vi "Ball and Beam(No Low Pass Fifter)2.vi"() -> ()   [LabVIEW 2011]
uses:
  <vilib>/Utility/file.llb/Write To Spreadsheet File (DBL).vi
  Instance           1 41Saved   Ball and Beam(No Low Pass Fifter) .vi
  Instance           2 41Saved   Ball and Beam(No Low Pass Fifter) .vi
panel:
  in  "file path (dialog if empty)":path
  out "Theta Output":dbl
  out "X Error":dbl
  out "X Error":dbl(graph)=-0.6885397082002527
  in  "Theta Bound":dbl=3.0
  in  "Kp":dbl=0.5
  in  "Kd":dbl
  in  "X disire":dbl
  out "Vout":dbl
  in  "Vout Bound":dbl=4.5
  in  "Kp1":dbl=1.0
  in  "Sampling rate(Hz)":dbl=50.0
  out "Theta":dbl
  in  "t offset":dbl
  in  "t amp":dbl
  out "Position":dbl
  in  "x offset":dbl
  in  "x amp":dbl
  out "Theta voltage":dbl
  out "X voltage":dbl
  in  "stop":bool
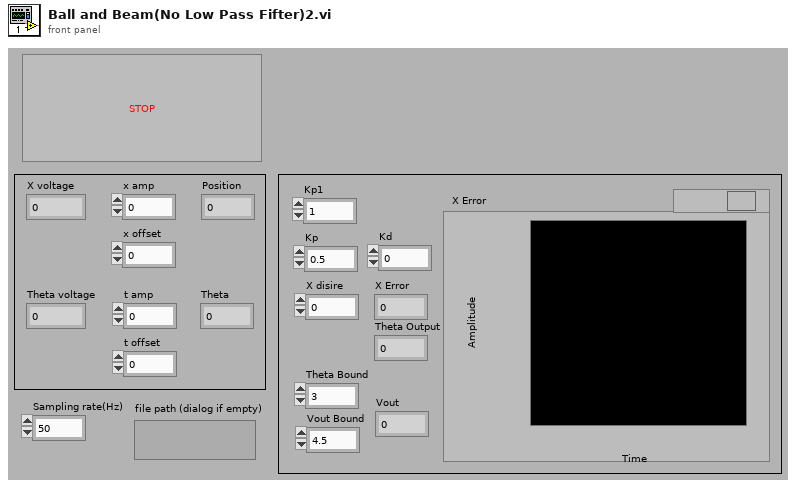
[diagram p1: front panel]
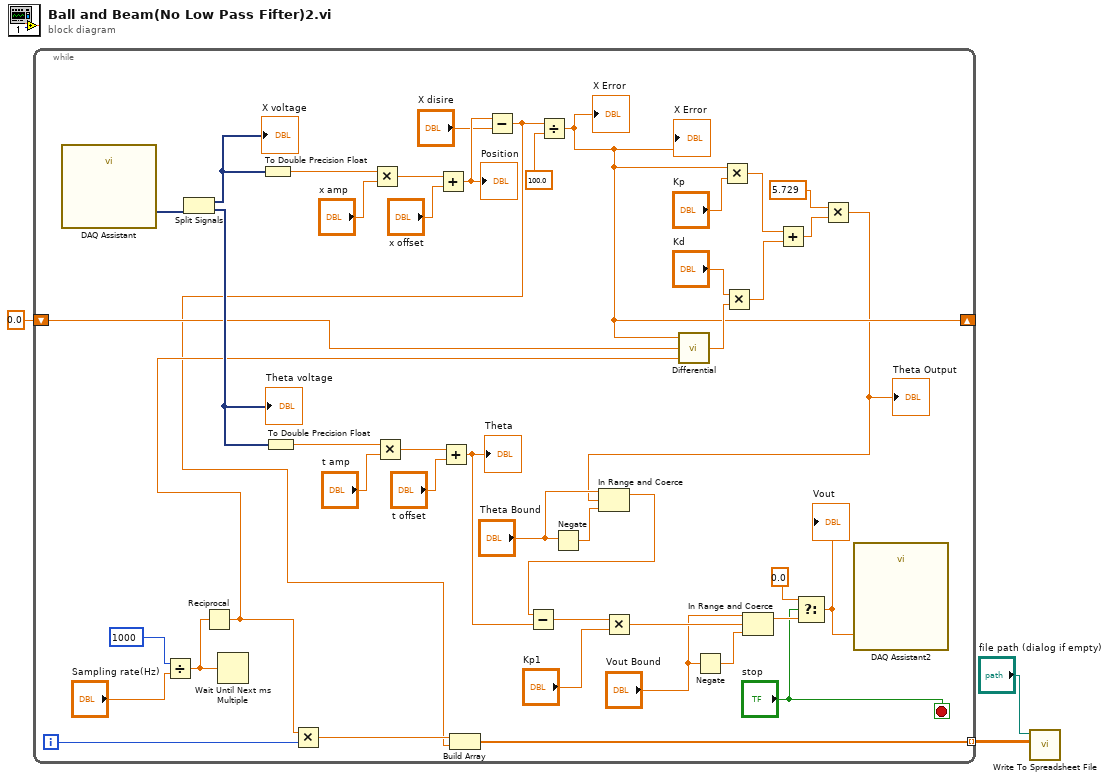
[diagram p0: block diagram]
diagram:
  n1 = while {
    shift-right: [w10] -> _
    shift-left: 0.0 -> [w19]
    tunnel: [w4] -> w2 mode=indexing
    i -> [w12]
    stop <- "stop" stop-if-true
    n2 = call "DAQ Assistant"() -> ("data"=w44:dynamicdata)  [unwired: 17 in, 2 out]
    n3 = Divide(x=1000, y="Sampling rate(Hz)") -> (x/y=w25:dbl)
    n4 = Split Signals(w44) -> (w43:dynamicdata, w38:dynamicdata)  [unwired: 2 in]
    "X voltage" <- w43
    "Theta voltage" <- w38
    n5 = Reciprocal(x=w25) -> (1/x=w11:dbl)
    n6 = Wait Until Next ms Multiple(millisecond multiple=w25) -> ()  [unwired: 1 out]
    n7 = To Double Precision Float(number=w43) -> (double precision float=w48:dbl)
    n8 = To Double Precision Float(number=w38) -> (double precision float=w42:dbl)
    n9 = Multiply(x=w11, y=w12) -> (x*y=w13:dbl)
    n10 = Multiply(x=w48, y="x amp") -> (x*y=w47:dbl)
    n11 = Multiply(x=w42, y="t amp") -> (x*y=w41:dbl)
    n12 = Add(x=w47, y="x offset") -> (x+y=w15:dbl)
    "Position" <- w15
    n13 = Add(x=w41, y="t offset") -> (x+y=w28:dbl)
    "Theta" <- w28
    n14 = Subtract(x=w15, y="X disire") -> (x-y=w5:dbl)
    n15 = Build Array(w13, w5) -> (w4:dbl[])
    n16 = Divide(x=w5, y=100.0) -> (x/y=w10:dbl)
    "X Error" <- w10
    "X Error" <- w10
    n17 = Negate(x="Theta Bound") -> (-x=w17:dbl)
    n18 = call "Differential.vi"("Ts"=w11, "X[k-1]"=w19, "X[k]"=w10) -> ("dX"=w24:dbl)
    n19 = Negate(x="Vout Bound") -> (-x=w33:dbl)
    n20 = Multiply(x=w10, y="Kp") -> (x*y=w21:dbl)
    n21 = Multiply(x="Kd", y=w24) -> (x*y=w20:dbl)
    n22 = Add(x=w21, y=w20) -> (x+y=w7:dbl)
    n23 = Multiply(x=5.729, y=w7) -> (x*y=w6:dbl)
    "Theta Output" <- w6
    n24 = In Range and Coerce(upper limit="Theta Bound", x=w6, lower limit=w17) -> (coerced(x)=w16:dbl)  [unwired: 1 out]
    n25 = Subtract(x=w16, y=w28) -> (x-y=w26:dbl)
    n26 = Multiply(x=w26, y="Kp1") -> (x*y=w32:dbl)
    n27 = In Range and Coerce(upper limit="Vout Bound", x=w32, lower limit=w33) -> (coerced(x)=w31:dbl)  [unwired: 1 out]
    n28 = Select(t=0.0, s="stop", f=w31) -> (s? t:f=w27:dbl)
    "Vout" <- w27
    n29 = call "DAQ Assistant2"("data"=w27) -> ()  [unwired: 17 in, 2 out]
  }
  n30 = call-poly <vilib>:"Write To Spreadsheet File.vi"("2D data"=w2, "file path (dialog if empty)"="file path (dialog if empty)") -> ()  [unwired: 6 in, 1 out]
